vi "Construct Base.vi"(8 "error in (no error)":errorcluster, 9 "channels":u8[](array[numeric]), 10 "identifier in":string, 11 "Execution Unit in (default object)":refnum<class "Execution Unit.lvclass">) -> (0 "error out":errorcluster, 3 "Execution Unit out":refnum<class "Execution Unit.lvclass">)   [LabVIEW 2020, in "AIM ARINC 429 Engine.lvlib" / "Implementation.lvlib" / "Execution Unit.lvclass"]
doc: "Creates a new Execution Unit object, or modifies all of the Execution Unit class properties of an existing Execution Unit object if an Execution Unit object is provided."
uses:
  Execution Unit.lvclass
  Execution Unit.lvclass/Execution Unit.ctl
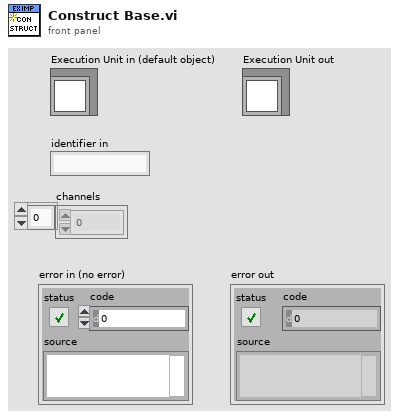
[diagram p1: front panel]
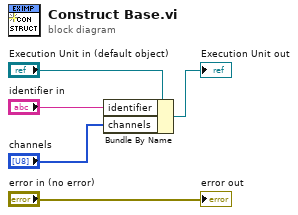
[diagram p0: block diagram]
diagram:
  n1 = Bundle By Name(cluster="Execution Unit in (default object)", "identifier"="identifier in", "channels"="channels") -> (→"Execution Unit out":refnum<class "Execution Unit.lvclass">)
  "error out" <- "error in (no error)"
